vi "AppLauncher.vi"   [LabVIEW 2023, in "AppLauncher.lvlib"]
uses:
  AppLauncher.lvlib
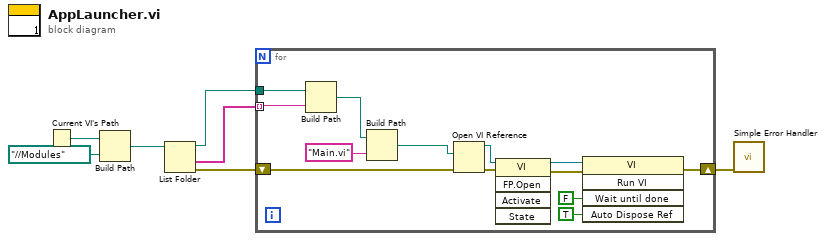
[diagram p0: block diagram]
diagram:
  n1 = Current VI's Path() -> (path=w7:path)
  n2 = Build Path(base path=w7, name or relative path=path "../../Modules") -> (appended path=w5:path)
  n3 = List Folder(path=w5) -> (path out=w3:path, folder names=w4:string[], error out=w2:errorcluster)  [unwired: 3 in, 1 out]
  n4 = for {
    tunnel: w4 -> [w19] mode=indexing
    tunnel: w3 -> [w20]
    shift-right: [w12] -> w1
    shift-left: w2 -> [w16]
    n5 = Build Path(base path=w20, name or relative path=w19) -> (appended path=w18:path)
    n6 = Build Path(base path=w18, name or relative path="Main.vi") -> (appended path=w15:path)
    n7 = Open VI Reference(vi path=w15, error in (no error)=w16) -> (vi reference=w10:refnum<vi>, error out=w11:errorcluster)  [unwired: 4 in]
    n8 = invoke class="VI" method="FP.Open"(reference=w10, error in=w11) -> (reference out=w9:refnum<vi>, error out=w8:errorcluster)  [unwired: 3 in, 3 out]
    n9 = invoke class="VI" method="Run VI"(reference=w9, error in=w8, "Wait until done"=FALSE ("Wait Until Done"), "Auto Dispose Ref"=TRUE ("Auto Dispose Reference")) -> (error out=w12:errorcluster)  [unwired: 1 in, 4 out]
  }
  n10 = call <vilib>:"Simple Error Handler.vi"("error in (no error)"=w1) -> ()  [unwired: 4 in, 5 out]
